vi "read.vi"(8 "error in (no error)":errorcluster, 10 "Stop Flag Reference":refnum<vi>, 11 "Photodiode in":refnum<class "Photodiode.lvclass">) -> (0 "error out":errorcluster, 3 "Photodiode out":refnum<class "Photodiode.lvclass">)   [LabVIEW 2014, in "Photodiode.lvclass"]
uses:
  Photodiode.lvclass
  Photodiode.lvclass/Photodiode.ctl
  <vilib>/DAQmx/read.llb/DAQmx Read (Analog 1D Wfm NChan NSamp).vi
  <vilib>/DAQmx/miscellaneous.llb/DAQmx Fill In Error Info.vi
panel:
  out "Elements In Data Queue":i32
  out "Elements In Display Queue":i32
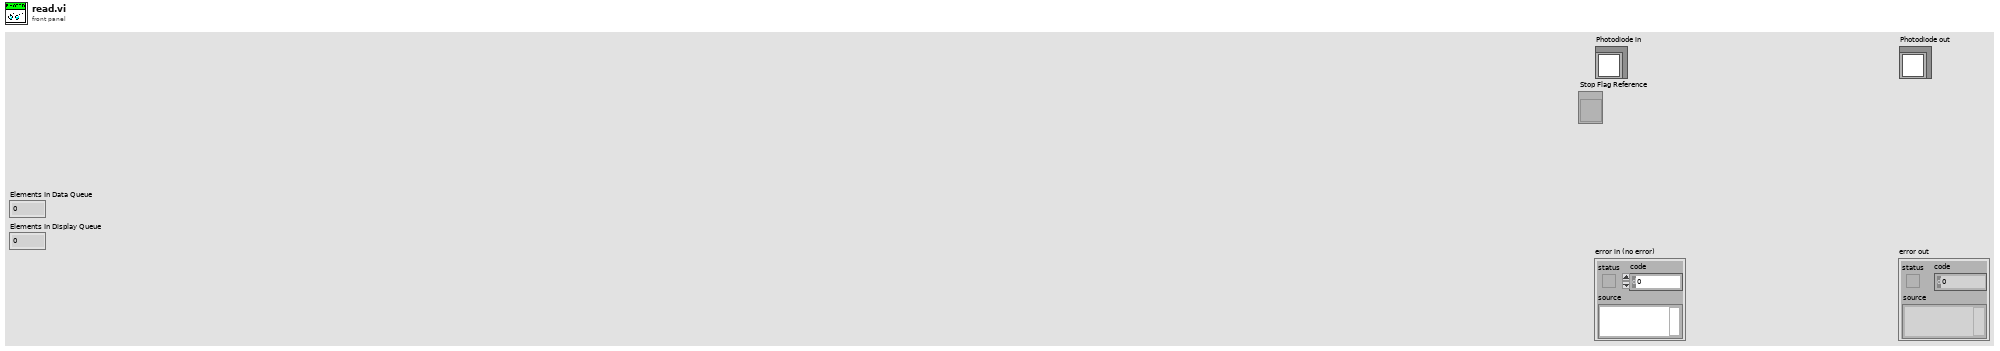
[diagram p1: front panel]
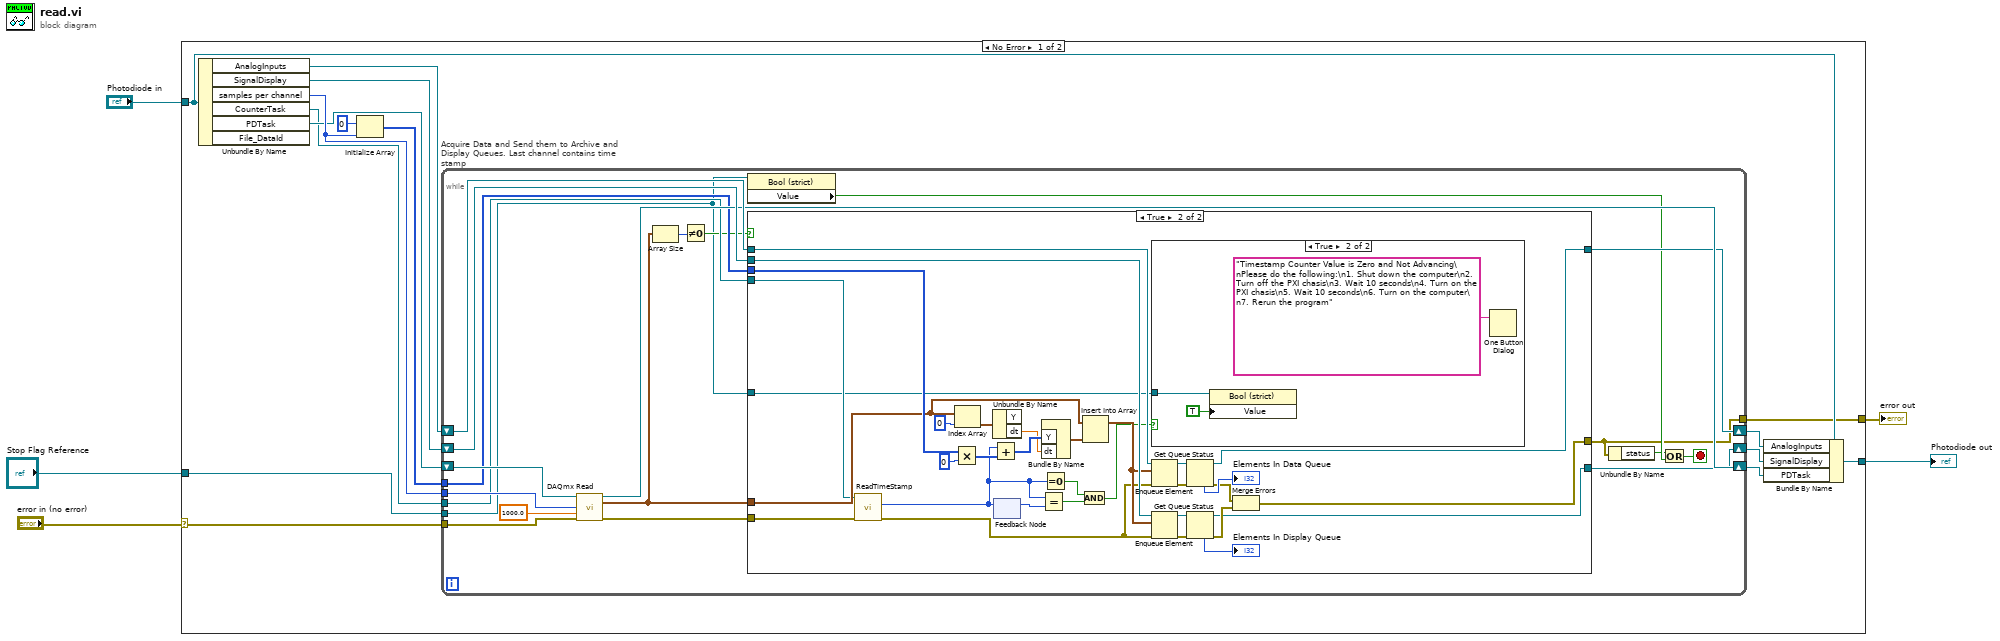
[diagram p0: block diagram]
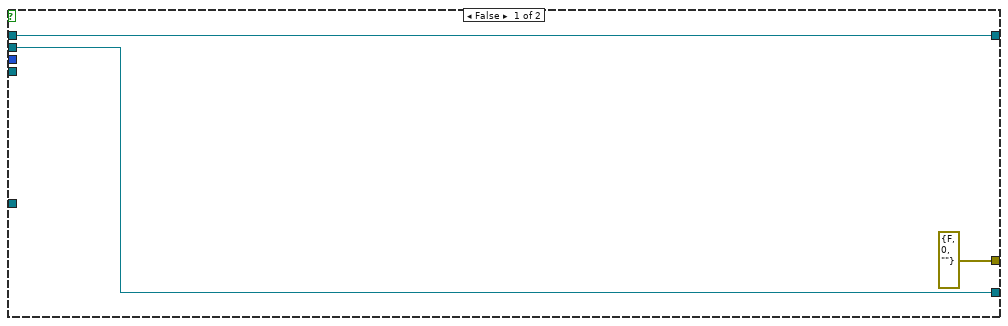
[diagram p2: hidden frame]
diagram:
  n1 = case shown="No Error" "error in (no error)" {
    selector: "error in (no error)" -> [w13 w80]
    tunnel: [w10 w80] -> w4
    tunnel: [w11 w79] -> w2
    tunnel: "Photodiode in" -> [w12 w79]
    tunnel: "Stop Flag Reference" -> [w6 _]
    frame No Error {
      n2 = Unbundle By Name(w12) -> ("AnalogInputs"=w14:refnum<queue>, "SignalDisplay"=w15:refnum<queue>, "samples per channel"=w18:i32, "CounterTask"=w16:refnum<k21>, "PDTask"=w17:refnum<k21>)  [unwired: 1 out]
      n3 = Initialize Array(u32 0 ("element"), w18) -> (w19:u32[])
      n4 = while "Acquire Data and Send them to Archive and Display Queues. Last channel contains time stamp" {
        tunnel: w13 -> [w39]
        tunnel: w18 -> [w38]
        shift-right: [w35] -> w9
        shift-left: w17 -> [w40]
        tunnel: [w29] -> w10
        tunnel: w16 -> [w33]
        tunnel: w19 -> [w34]
        shift-right: [w32] -> w7
        shift-left: w14 -> [w37]
        shift-right: [w31] -> w8
        shift-left: w15 -> [w36]
        tunnel: w6 -> [w21]
        stop <- w27 stop-if-true
        n5 = call-poly <vilib>:"DAQmx Read.vi"("task/channels in"=w40, "number of samples per channel"=w38, "timeout"=1000.0, "error in"=w39) -> ("task out"=w35:refnum<k21>, "data"=w26:waveform(dbl)[], "error out"=w25:errorcluster)  [unwired: 9 in]
        n6 = Array Size(array=w26) -> (size(s)=w24:i32)
        n7 = Not Equal To 0?(x=w24) -> (x != 0?=w23:bool)
        n8 = property class="Bool (strict)"(reference=w21) -> ("Value"=w30:bool)  [unwired: 1 in, 2 out]
        n9 = case shown="True" w23 {
          tunnel: w37 -> [w43 w75]
          tunnel: w36 -> [w42 w74]
          tunnel: w34 -> [_ w65]
          tunnel: w26 -> [_ w59]
          tunnel: [errorcluster {"status"=FALSE, "code"=0, "source"=""} ("error IO") w56] -> w29
          tunnel: w33 -> [_ w55]
          tunnel: [w43 w53] -> w32
          tunnel: [w42 w52] -> w31
          tunnel: w25 -> [_ w45]
          tunnel: w21 -> [_ w44]
          frame False {
          }
          frame True {
            n10 = call "ReadTimeStamp.vi"("error in"=w45, "task/channels in"=w55) -> ("error out"=w54:errorcluster, "data"=w51:u32)  [unwired: 7 in, 1 out]
            n11 = Multiply(x=w65, y=0) -> (x*y=w64:u32[])
            n12 = Index Array(array=w59, index=0) -> (element=w61:waveform(dbl))
            n13 = Unbundle By Name(w61) -> ("dt"=w60:dbl)  [unwired: 1 out]
            n14 = Add(x=w51, y=w64) -> (x+y=w63:u32[])
            n15 = feedback #1() -> (w50:u32)  [unwired: 1 in]
            n16 = feedback-in #1(w51) -> ()
            n17 = Equal?(x=w51, y=w50) -> (x = y?=w48:bool)
            n18 = Bundle By Name("Y"=w63, "dt"=w60) -> (w58:waveform(u32))  [unwired: 1 in]
            n19 = Equal To 0?(x=w51) -> (x = 0?=w49:bool)
            n20 = And(x=w49, y=w48) -> (x .and. y?=w47:bool)
            n21 = Insert Into Array(array=w59, new element=w58) -> (w57:waveform(dbl)[])  [unwired: 1 in]
            n22 = case shown="True" w47 {
              tunnel: w44 -> [_ w76]
              frame False {
              }
              frame True {
                n23 = property class="Bool (strict)"(reference=w76, "Value"=TRUE) -> ()  [unwired: 1 in, 2 out]
                n24 = One Button Dialog(message="Timestamp Counter Value is Zero and Not Advancing\nPlease do the following:\n1. Shut down the computer\n2. Turn off the PXI chasis\n3. Wait 10 seconds\n4. Turn on the PXI chasis\n5. Wait 10 seconds\n6. Turn on the computer\n7. Rerun the program") -> ()  [unwired: 1 in, 1 out]
              }
            }
            n25 = Enqueue Element(queue=w75, element=w57, error in (no error)=w54) -> (queue out=w73:refnum<queue>, error out=w70:errorcluster)  [unwired: 1 in, 1 out]
            n26 = Enqueue Element(queue=w74, element=w57, error in (no error)=w54) -> (queue out=w71:refnum<queue>, error out=w69:errorcluster)  [unwired: 1 in, 1 out]
            n27 = Get Queue Status(queue=w73, error in (no error)=w70) -> (queue out=w53:refnum<queue>, error out=w68:errorcluster, # elements in queue=→"Elements In Data Queue":i32)  [unwired: 1 in, 5 out]
            n28 = Get Queue Status(queue=w71, error in (no error)=w69) -> (queue out=w52:refnum<queue>, error out=w67:errorcluster, # elements in queue=→"Elements In Display Queue":i32)  [unwired: 1 in, 5 out]
            n29 = Merge Errors(w68, w67) -> (w56:errorcluster)
          }
        }
        n30 = Unbundle By Name(w29) -> ("status"=w28:bool)
        n31 = Or(x=w28, y=w30) -> (x .or. y?=w27:bool)
      }
      n32 = Bundle By Name(cluster=w12, "AnalogInputs"=w7, "SignalDisplay"=w8, "PDTask"=w9) -> (w11:refnum<class "Photodiode.lvclass">)
    }
    frame Error {
    }
  }
  "error out" <- w4
  "Photodiode out" <- w2
